vi "Run_Wavedump.vi"(6 "Close":bool, 7 "Start":bool, 8 "Channel":string[](array[string]), 9 "PMTs":string[](array[string]), 11 "Test":string(combo)) -> (0 "Error":string="\n", 1 "Event Build Error":bool, 2 "Over Temperature":bool, 3 "Command Line Output":string)   [LabVIEW 2018]
panel:
  in  "Tab Control":enum32{"Controls", "Read Me"}(tab)
  out "Wait Completed":bool
  out "Waited to Copy Files (s)":u32
  out "Wait to Copy  Files (s)":u32=20
  out "Bash Script Run":bool=TRUE
  in  "View PMT Files":bool
  # "This application is used to send a command to run the bash script relating to an electrical test for PMTs. The bash script will run wavedump in a preset configuration.\n\nUse the Controls tab to send the necessary commands.\n\nTo run, enter up to 8 PMT numbers and the channels they are connected to on the digitiser.\n\nSelect the test to run and press \"Start\".\n\nA window will pop up to display the waveform as it is being recorded.\n\nTo view other PMT files or scroll through the ones being recorded, press \"View PMT Files\".\n\nAs the program only sends a command, it can't be used to stop or control wavedump.\n\nPress \"CLOSE\" to close the application."
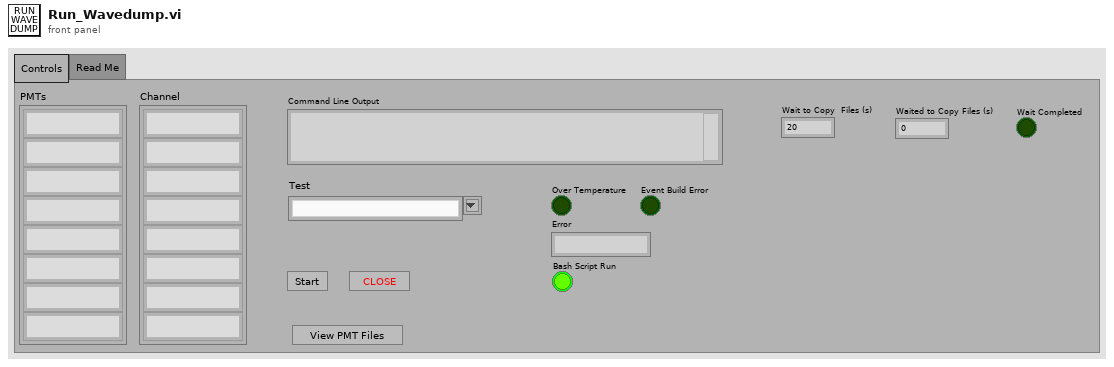
[diagram p1: front panel]
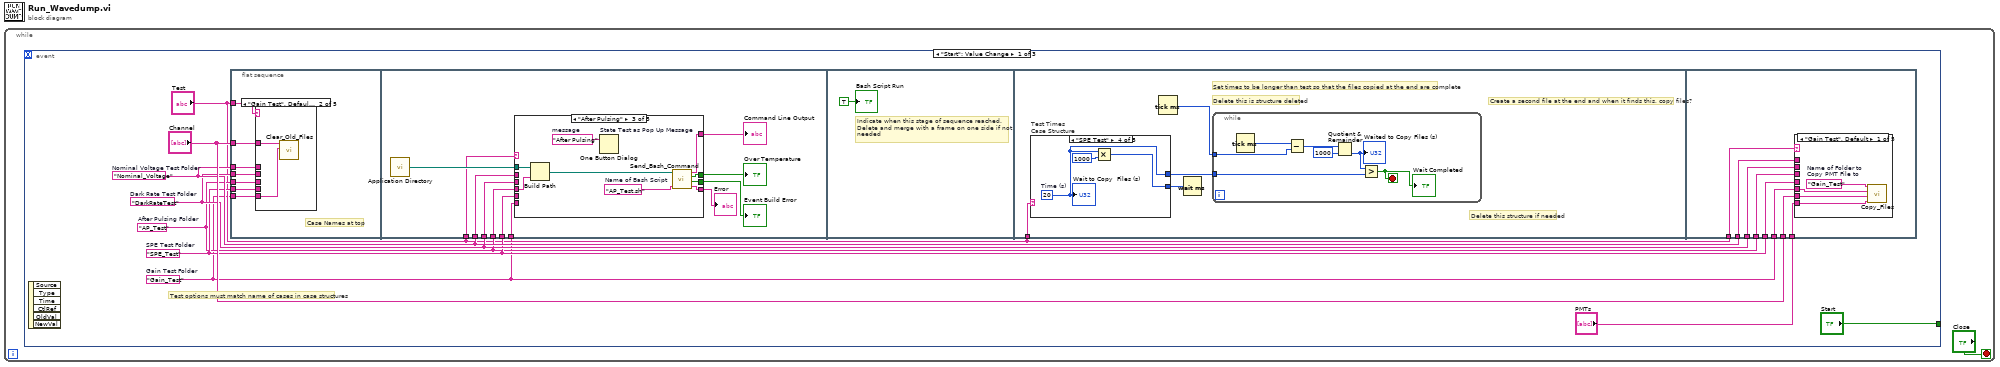
[diagram p0: block diagram]
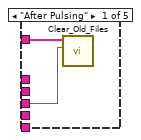
[diagram p2: hidden frame]
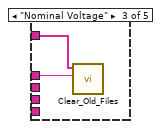
[diagram p3: hidden frame]
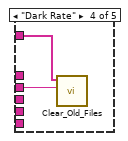
[diagram p4: hidden frame]
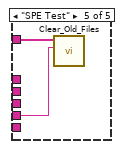
[diagram p5: hidden frame]
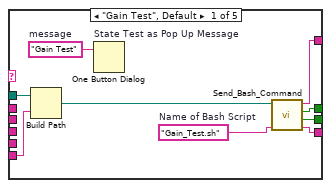
[diagram p6: hidden frame]
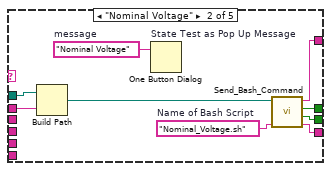
[diagram p7: hidden frame]
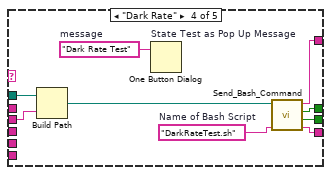
[diagram p8: hidden frame]
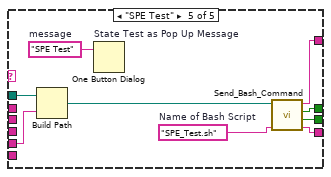
[diagram p9: hidden frame]
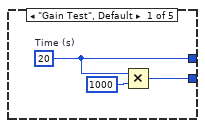
[diagram p10: hidden frame]
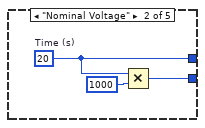
[diagram p11: hidden frame]
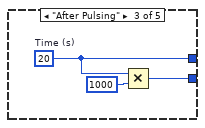
[diagram p12: hidden frame]
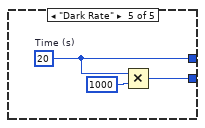
[diagram p13: hidden frame]
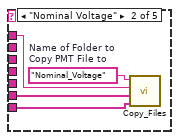
[diagram p14: hidden frame]
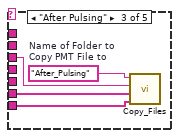
[diagram p15: hidden frame]
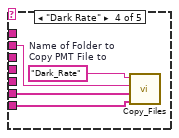
[diagram p16: hidden frame]
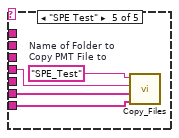
[diagram p17: hidden frame]
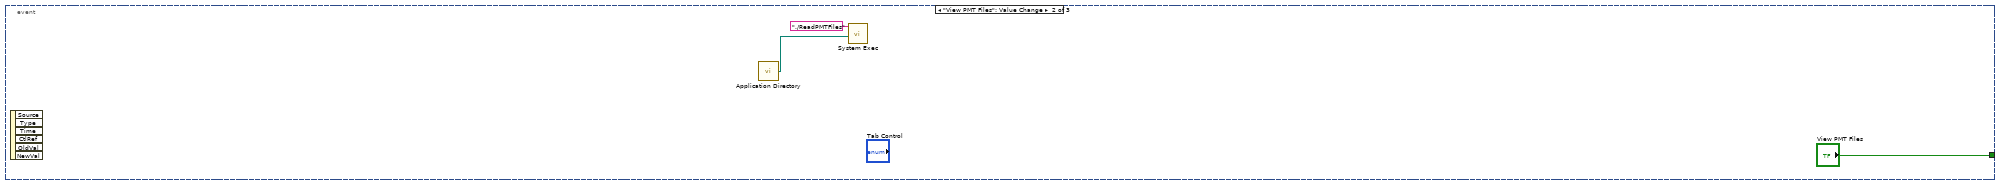
[diagram p18: hidden frame]
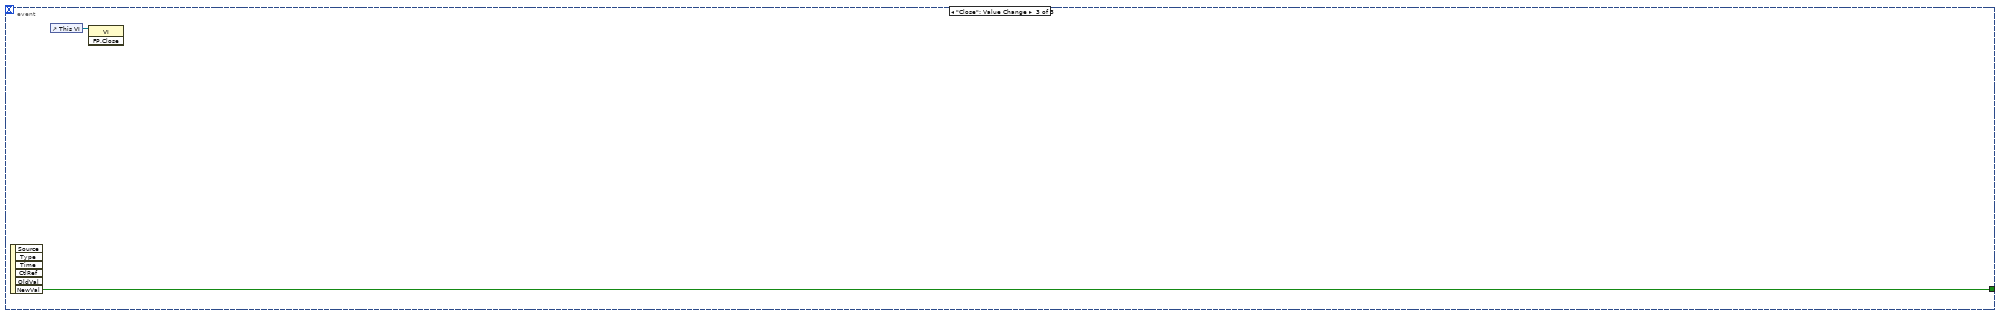
[diagram p19: hidden frame]
diagram:
  n1 = while {
    stop <- "Close" stop-if-true
    n2 = event shown="[0] \"Start\": Value Change" {
      selector: _ -> [_ _ _]
      dyn-events: _ -> [_ _ _]
      timeout: _ -> [_ _ _]
      tunnel: ["Start" "View PMT Files" w143] -> _
      event "Start": Value Change {
        w4 = "AP_Test"  # After Pulsing Folder
        w6 = "DarkRateTest"  # Dark Rate Test Folder
        w5 = "SPE_Test"  # SPE Test Folder
        w7 = "Nominal_Voltage"  # Nominal Voltage Test Folder
        w2 = "Gain_Test"  # Gain Test Folder
        # "Test options must match name of cases in case structures"
        n3 = event-data() -> ()  [unwired: 1 in, 6 out]
        n4 = flat-sequence {
          tunnel: "Channel" -> [w17]
          tunnel: "Test" -> [w16]
          tunnel: w7 -> [w15]
          tunnel: w6 -> [w14]
          tunnel: w5 -> [w13]
          tunnel: w4 -> [w12]
          tunnel: w2 -> [w11]
          tunnel: "Test" -> [w33]
          tunnel: w2 -> [w32]
          tunnel: w7 -> [w31]
          tunnel: w5 -> [w30]
          tunnel: w6 -> [w29]
          tunnel: w4 -> [w28]
          tunnel: "Test" -> [w87]
          tunnel: "PMTs" -> [w115]
          tunnel: "Test" -> [w118]
          tunnel: w4 -> [w117]
          tunnel: "Channel" -> [w116]
          tunnel: w6 -> [w114]
          tunnel: w5 -> [w113]
          tunnel: w2 -> [w112]
          tunnel: w7 -> [w111]
          frame #0 {
            # "Case Names at top"
            n5 = case shown="\"Gain Test\", Default" w16 {
              tunnel: w17 -> [w19 w21 w23 w25 w27]
              tunnel: w15 -> [_ _ w22 _ _]
              tunnel: w14 -> [_ _ _ w24 _]
              tunnel: w13 -> [_ _ _ _ w26]
              tunnel: w12 -> [w18 _ _ _ _]
              tunnel: w11 -> [_ w20 _ _ _]
              frame "After Pulsing" {
                n6 = call "Clear_Old_Files.vi"("Bash Script Folder Name"=w18, "Channel"=w19) -> ()  [unwired: 10 in]
              }
              frame "Gain Test", Default {
                n7 = call "Clear_Old_Files.vi"("Bash Script Folder Name"=w20, "Channel"=w21) -> ()  [unwired: 10 in]
              }
              frame "Nominal Voltage" {
                n8 = call "Clear_Old_Files.vi"("Bash Script Folder Name"=w22, "Channel"=w23) -> ()  [unwired: 10 in]
              }
              frame "Dark Rate" {
                n9 = call "Clear_Old_Files.vi"("Bash Script Folder Name"=w24, "Channel"=w25) -> ()  [unwired: 10 in]
              }
              frame "SPE Test" {
                n10 = call "Clear_Old_Files.vi"("Bash Script Folder Name"=w26, "Channel"=w27) -> ()  [unwired: 10 in]
              }
            }
          }
          frame #1 {
            n11 = call <vilib>:"Application Directory.vi"() -> ("Application Directory"=w38:path)
            n12 = case shown="\"After Pulsing\"" w33 {
              tunnel: [w39 w48 w57 w66 w75] -> w34
              tunnel: [w40 w49 w58 w67 w76] -> w35
              tunnel: [w41 w50 w59 w68 w77] -> w36
              tunnel: [w42 w51 w60 w69 w78] -> w37
              tunnel: w38 -> [w44 w53 w61 w72 w80]
              tunnel: w32 -> [w43 _ _ _ _]
              tunnel: w31 -> [_ w52 _ _ _]
              tunnel: w30 -> [_ _ _ _ w79]
              tunnel: w29 -> [_ _ _ w70 _]
              tunnel: w28 -> [_ _ w62 _ _]
              frame "Gain Test", Default {
                w46 = "Gain Test"  # message
                w47 = "Gain_Test.sh"  # Name of Bash Script
                n13 = Build Path(base path=w44, name or relative path=w43) -> (appended path=w45:path)
                n14 = One Button Dialog "State Test as Pop Up Message"(message=w46) -> ()  [unwired: 1 in, 1 out]
                n15 = call "Send_Bash_Command.vi"("working directory"=w45, "Bash script"=w47) -> ("Command Line Output"=w42:string, "Over Temperature"=w41:bool, "Event Build Error"=w40:bool, "Error"=w39:string)  [unwired: 5 in]
              }
              frame "Nominal Voltage" {
                w55 = "Nominal Voltage"  # message
                w56 = "Nominal_Voltage.sh"  # Name of Bash Script
                n16 = Build Path(base path=w53, name or relative path=w52) -> (appended path=w54:path)
                n17 = One Button Dialog "State Test as Pop Up Message"(message=w55) -> ()  [unwired: 1 in, 1 out]
                n18 = call "Send_Bash_Command.vi"("working directory"=w54, "Bash script"=w56) -> ("Command Line Output"=w51:string, "Over Temperature"=w50:bool, "Event Build Error"=w49:bool, "Error"=w48:string)  [unwired: 5 in]
              }
              frame "After Pulsing" {
                w64 = "After Pulsing"  # message
                w65 = "AP_Test.sh"  # Name of Bash Script
                n19 = Build Path(base path=w61, name or relative path=w62) -> (appended path=w63:path)
                n20 = One Button Dialog "State Test as Pop Up Message"(message=w64) -> ()  [unwired: 1 in, 1 out]
                n21 = call "Send_Bash_Command.vi"("working directory"=w63, "Bash script"=w65) -> ("Command Line Output"=w60:string, "Over Temperature"=w59:bool, "Event Build Error"=w58:bool, "Error"=w57:string)  [unwired: 5 in]
              }
              frame "Dark Rate" {
                w74 = "Dark Rate Test"  # message
                w71 = "DarkRateTest.sh"  # Name of Bash Script
                n22 = Build Path(base path=w72, name or relative path=w70) -> (appended path=w73:path)
                n23 = One Button Dialog "State Test as Pop Up Message"(message=w74) -> ()  [unwired: 1 in, 1 out]
                n24 = call "Send_Bash_Command.vi"("working directory"=w73, "Bash script"=w71) -> ("Command Line Output"=w69:string, "Over Temperature"=w68:bool, "Event Build Error"=w67:bool, "Error"=w66:string)  [unwired: 5 in]
              }
              frame "SPE Test" {
                w82 = "SPE Test"  # message
                w83 = "SPE_Test.sh"  # Name of Bash Script
                n25 = Build Path(base path=w80, name or relative path=w79) -> (appended path=w81:path)
                n26 = One Button Dialog "State Test as Pop Up Message"(message=w82) -> ()  [unwired: 1 in, 1 out]
                n27 = call "Send_Bash_Command.vi"("working directory"=w81, "Bash script"=w83) -> ("Command Line Output"=w78:string, "Over Temperature"=w77:bool, "Event Build Error"=w76:bool, "Error"=w75:string)  [unwired: 5 in]
              }
            }
            "Command Line Output" <- w37
            "Over Temperature" <- w36
            "Event Build Error" <- w35
            "Error" <- w34
          }
          frame #2 {
            # "Indicate when this stage of sequence reached.\nDelete and merge with a frame on one side if not needed"
            "Bash Script Run" <- TRUE
          }
          frame #3 {
            # "Create a second file at the end and when it finds this, copy files?"
            # "Delete this is structure deleted"
            # "Delete this structure if needed"
            # "Set times to be longer than test so that the files copied at the end are complete"
            n28 = case "Test Times\nCase Structure" shown="\"SPE Test\"" w87 {
              tunnel: [w97 w100 w103 w106 w110] -> w88
              tunnel: [w96 w99 w102 w105 w108] -> w85
              frame "Gain Test", Default {
                w96 = u32 20  # Time (s)
                n29 = Multiply(x=w96, y=u32 1000) -> (x*y=w97:u32)
              }
              frame "Nominal Voltage" {
                w99 = u32 20  # Time (s)
                n30 = Multiply(x=w99, y=u32 1000) -> (x*y=w100:u32)
              }
              frame "After Pulsing" {
                w102 = u32 20  # Time (s)
                n31 = Multiply(x=w102, y=u32 1000) -> (x*y=w103:u32)
              }
              frame "SPE Test" {
                w105 = u32 20  # Time (s)
                n32 = Multiply(x=w105, y=u32 1000) -> (x*y=w106:u32)
                "Wait to Copy  Files (s)" <- w105
              }
              frame "Dark Rate" {
                w108 = u32 20  # Time (s)
                n33 = Multiply(x=w108, y=u32 1000) -> (x*y=w110:u32)
              }
            }
            n34 = Tick Count (ms)() -> (millisecond timer value=w86:u32)
            n35 = Wait (ms)(milliseconds to wait=w88) -> ()  [unwired: 1 out]
            n36 = while {
              tunnel: w86 -> [w94]
              tunnel: w85 -> [w90]
              stop <- w89 stop-if-true
              n37 = Tick Count (ms)() -> (millisecond timer value=w95:u32)
              n38 = Subtract(x=w95, y=w94) -> (x-y=w93:u32)
              n39 = Quotient & Remainder(x=w93, y=u32 1000) -> (floor(x/y)=w91:u32)  [unwired: 1 out]
              "Waited to Copy Files (s)" <- w91
              n40 = Greater?(x=w91, y=w90) -> (0:w89:bool)
              "Wait Completed" <- w89
            }
          }
          frame #4 {
            n41 = case shown="\"Gain Test\", Default" w118 {
              tunnel: w117 -> [_ _ w130 _ _]
              tunnel: w116 -> [w120 w124 w128 w132 w136]
              tunnel: w115 -> [w119 w123 w127 w131 w135]
              tunnel: w114 -> [_ _ _ w133 _]
              tunnel: w113 -> [_ _ _ _ w137]
              tunnel: w112 -> [w121 _ _ _ _]
              tunnel: w111 -> [_ w125 _ _ _]
              frame "Gain Test", Default {
                w122 = "Gain_Test"  # Name of Folder to Copy PMT File to
                n42 = call "Copy_Files.vi"("PMTs"=w119, "Channel"=w120, "Folder Containing Bash Script"=w121, "Name of Folder to\nCopy PMT File to"=w122) -> ()  [unwired: 8 in]
              }
              frame "Nominal Voltage" {
                w126 = "Nominal_Voltage"  # Name of Folder to Copy PMT File to
                n43 = call "Copy_Files.vi"("PMTs"=w123, "Channel"=w124, "Folder Containing Bash Script"=w125, "Name of Folder to\nCopy PMT File to"=w126) -> ()  [unwired: 8 in]
              }
              frame "After Pulsing" {
                w129 = "After_Pulsing"  # Name of Folder to Copy PMT File to
                n44 = call "Copy_Files.vi"("PMTs"=w127, "Channel"=w128, "Folder Containing Bash Script"=w130, "Name of Folder to\nCopy PMT File to"=w129) -> ()  [unwired: 8 in]
              }
              frame "Dark Rate" {
                w134 = "Dark_Rate"  # Name of Folder to Copy PMT File to
                n45 = call "Copy_Files.vi"("PMTs"=w131, "Channel"=w132, "Folder Containing Bash Script"=w133, "Name of Folder to\nCopy PMT File to"=w134) -> ()  [unwired: 8 in]
              }
              frame "SPE Test" {
                w138 = "SPE_Test"  # Name of Folder to Copy PMT File to
                n46 = call "Copy_Files.vi"("PMTs"=w135, "Channel"=w136, "Folder Containing Bash Script"=w137, "Name of Folder to\nCopy PMT File to"=w138) -> ()  [unwired: 8 in]
              }
            }
          }
        }
      }
      event "View PMT Files": Value Change {
        n47 = event-data() -> ()  [unwired: 1 in, 6 out]
        n48 = call <vilib>:"Application Directory.vi"() -> ("Application Directory"=w139:path)
        n49 = call <vilib>:"System Exec.vi"("working directory"=w139, "command line"="./ReadPMTFiles") -> ()  [unwired: 6 in, 4 out]
      }
      event "Close": Value Change {
        n50 = event-data() -> ("NewVal"=w143:bool)  [unwired: 1 in, 5 out]
        n51 = control-ref of="This VI"() -> (w142:refnum<vi>)
        n52 = invoke class="VI" method="FP.Close"(reference=w142) -> ()  [unwired: 2 in, 3 out]
      }
    }
  }
